vi "ATS_Check.vi"(9 "ATS_Check":T1, 10 "BoardToVerify":string, 11 "Device":i32) -> (1 "OK":bool, 3 "DeviceOut":i32)   [LabVIEW 2015]
doc: "_____AlazarTech, Scope_____\n\nCheck compatibility with the selected Board.\n\nInput:\n'NONE': no limitation\n'NO ATS9462' : ATS9462 cannot run in this application.\n'ATS9462_Traditional' : ATS9462 cannot run in traditional mode.\n'OnBoard Memory': need memory on the device to continue. \n\n\nOutput:\n\n`OK`: no problem found."
uses:
  ATS_ctl/ATS_Check_Ctrl.ctl
  ATS_ctl/ATS_Global_Ctrl.ctl
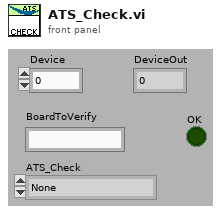
[diagram p1: front panel]
types:
  T1 = typedef "ATS_Check_Ctrl.ctl" = enum16{"None", "NO_ATS9462", "ATS9462_Traditional", "Verify Board", "OnBoard Memory", "Board & Memory", "Master/Slave", "NO Master/Slave"}
  T2 = typedef "ATS_Global_Ctrl.ctl" = enum16{"Init_Device", "Clear_ALL", "Set", "Get"}
  T3 = typedef "Device_Info.ctl" = cluster{"Handle":u32, "Board":string, "CPLD":string, "MemorySize":u32, "SampleSize":u8, "ID":i32, "High_Memory":bool, "Chan/Board":u8}
  T4 = typedef "ATS_Sys_Info.ctl" = cluster{"MS_Mode":bool, "MBoard":i32, "#Board":i32}
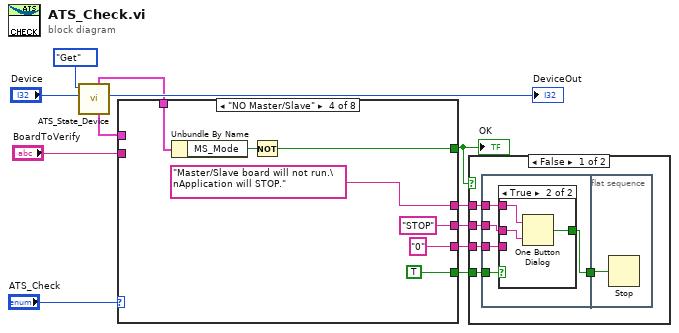
[diagram p0: block diagram]
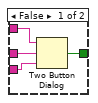
[diagram p2: hidden frame]
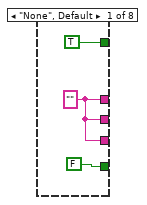
[diagram p4: hidden frame]
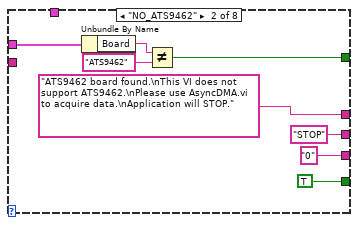
[diagram p5: hidden frame]
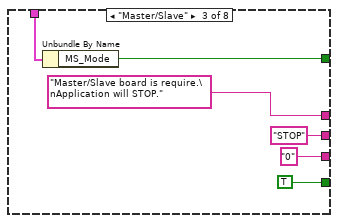
[diagram p6: hidden frame]
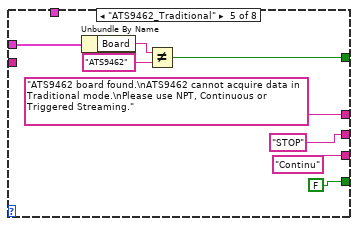
[diagram p7: hidden frame]
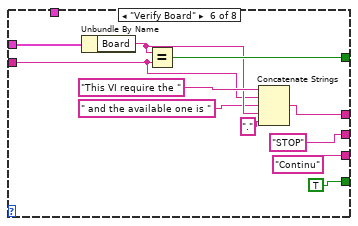
[diagram p8: hidden frame]
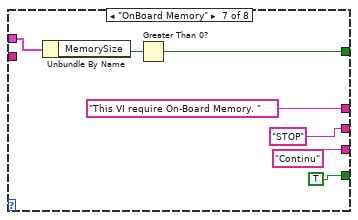
[diagram p9: hidden frame]
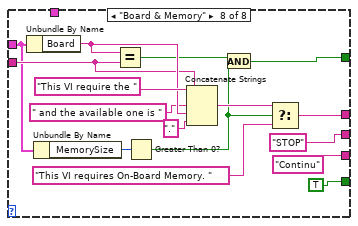
[diagram p10: hidden frame]
diagram:
  n1 = call "ATS_State_Device.vi"("DeviceIn"="Device", "ATS_GBL_Ctrl"=ATS_Global_Ctrl."Get") -> ("DeviceOut"=→"DeviceOut":i32, "DevInfo_Out"=w9:T3, "Sys_Out"=w1:T4)  [unwired: 4 in, 3 out]
  n2 = case shown="\"NO Master/Slave\"" "ATS_Check" {
    tunnel: w9 -> [_ w23 _ _ w44 w55 w62 w70]
    tunnel: [TRUE w20 w24 w30 w41 w54 w57 w64] -> w7
    tunnel: [w13 "ATS9462 board found.\nThis VI does not support ATS9462.\nPlease use AsyncDMA.vi to acquire data.\nApplication will STOP." ("message") "Master/Slave board is require.\nApplication will STOP." ("message") "Master/Slave board will not run.\nApplication will STOP." ("message") "ATS9462 board found.\nATS9462 cannot acquire data in Traditional mode.\nPlease use NPT, Continuous or Triggered Streaming." ("message") w46 "This VI require On-Board Memory. " ("message") w68] -> w6
    tunnel: [w13 "0" ("message") "0" ("message") "0" ("message") "Continu" ("message") "Continu" ("message") "Continu" ("message") "Continu" ("message")] -> w5
    tunnel: [FALSE ("stop? (T)") TRUE ("stop? (T)") TRUE ("stop? (T)") TRUE ("stop? (T)") FALSE ("stop? (T)") TRUE ("stop? (T)") TRUE ("stop? (T)") TRUE ("stop? (T)")] -> w4
    tunnel: [w13 "STOP" ("message") "STOP" ("message") "STOP" ("message") "STOP" ("message") "STOP" ("message") "STOP" ("message") "STOP" ("message")] -> w3
    tunnel: "BoardToVerify" -> [_ _ _ _ _ w45 _ w71]
    tunnel: w1 -> [_ _ w25 w32 _ _ _ _]
    frame "None", Default {
      w13 = "" ("message")
    }
    frame "NO_ATS9462" {
      n3 = Unbundle By Name(w23) -> ("Board"=w22:string)
      n4 = Not Equal?(x=w22, y="ATS9462") -> (x != y?=w20:bool)
    }
    frame "Master/Slave" {
      n5 = Unbundle By Name(w25) -> ("MS_Mode"=w24:bool)
    }
    frame "NO Master/Slave" {
      n6 = Unbundle By Name(w32) -> ("MS_Mode"=w31:bool)
      n7 = Not(x=w31) -> (.not. x?=w30:bool)
    }
    frame "ATS9462_Traditional" {
      n8 = Unbundle By Name(w44) -> ("Board"=w43:string)
      n9 = Not Equal?(x=w43, y="ATS9462") -> (x != y?=w41:bool)
    }
    frame "Verify Board" {
      n10 = Unbundle By Name(w55) -> ("Board"=w49:string)
      n11 = Equal?(x=w49, y=w45) -> (x = y?=w54:bool)
      n12 = Concatenate Strings("This VI require the " ("message"), w45, " and the available one is " ("string"), w49, "." ("string")) -> (w46:string)
    }
    frame "OnBoard Memory" {
      n13 = Unbundle By Name(w62) -> ("MemorySize"=w58:u32)
      n14 = Greater Than 0?(x=w58) -> (x > 0?=w57:bool)
    }
    frame "Board & Memory" {
      n15 = Unbundle By Name(w70) -> ("Board"=w74:string)
      n16 = Unbundle By Name(w70) -> ("MemorySize"=w63:u32)
      n17 = Equal?(x=w74, y=w71) -> (x = y?=w65:bool)
      n18 = Greater Than 0?(x=w63) -> (x > 0?=w66:bool)
      n19 = Concatenate Strings("This VI require the " ("message"), w71, " and the available one is " ("string"), w74, "." ("string")) -> (w67:string)
      n20 = And(x=w65, y=w66) -> (x .and. y?=w64:bool)
      n21 = Select(t=w67, s=w66, f="This VI requires On-Board Memory. " ("message")) -> (s? t:f=w68:string)
    }
  }
  "OK" <- w7
  n22 = case shown="False" w7 {
    tunnel: w6 -> [w83 _]
    tunnel: w5 -> [w82 _]
    tunnel: w4 -> [w81 _]
    tunnel: w3 -> [w79 _]
    frame False {
      n23 = flat-sequence {
        tunnel: w83 -> [w88]
        tunnel: w82 -> [w87]
        tunnel: w81 -> [w84]
        tunnel: [w86] -> w80
        tunnel: w79 -> [w85]
        tunnel: w80 -> [w96]
        frame #0 {
          n24 = case shown="True" w84 {
            tunnel: w88 -> [w92 w94]
            tunnel: w87 -> [w91 _]
            tunnel: [w90 w95] -> w86
            tunnel: w85 -> [w89 w93]
            frame False {
              n25 = Two Button Dialog(message=w92, 1:w91, 2:w89) -> (T button?=w90:bool)
            }
            frame True {
              n26 = One Button Dialog(message=w94, button name ("OK")=w93) -> (true=w95:bool)
            }
          }
        }
        frame #1 {
          n27 = Stop(stop? (T)=w96) -> ()
        }
      }
    }
    frame True {
    }
  }
